vi "Limelight HatchPanel.vi"(7 "Max Speed":dbl=0.6, 8 "error in":errorcluster, 10 "Max Time ms (2000)":u32=2000, 11 "Min time ms (500)":u32=500) -> (0 "error out":errorcluster, 3 "Timed Out?":bool)   [LabVIEW 2018]
uses:
  <vilib>/Rock Robotics/Network Tables/NT Read Number.vi
  Auton Kill Switch.vi
panel:
  in  "allowed error":dbl=2.5
  in  "kpDist":dbl=0.2
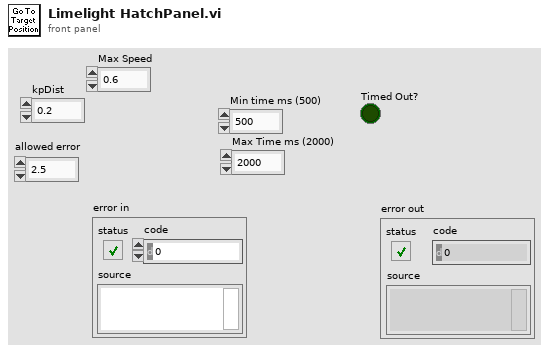
[diagram p1: front panel]
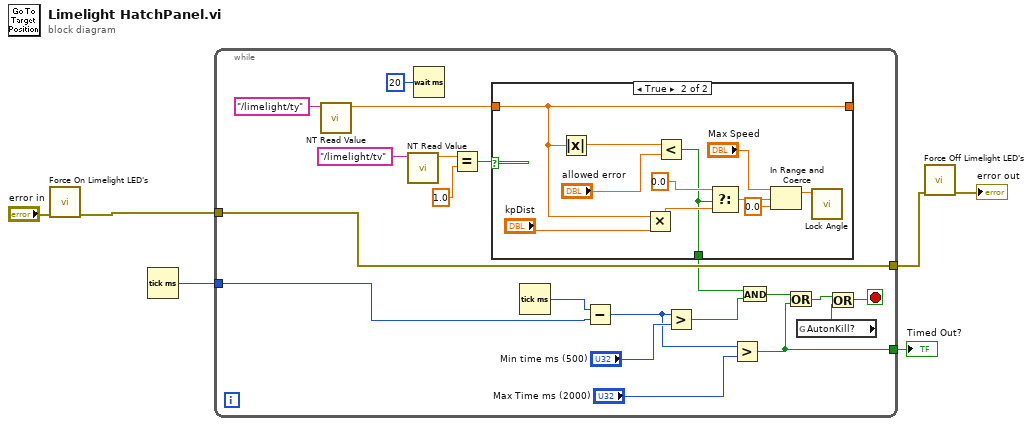
[diagram p0: block diagram]
diagram:
  n1 = call "Force On Limelight LED's.vi"("error in"="error in") -> ("error out"=w5:errorcluster)  [unwired: 9 in]
  n2 = Tick Count (ms)() -> (millisecond timer value=w2:u32)
  n3 = while {
    tunnel: w5 -> [w19]
    tunnel: [w19] -> w4
    tunnel: w2 -> [w17]
    tunnel: [w9] -> w1
    stop <- w8 stop-if-true
    n4 = call-poly <vilib>:"NT Read Value.vi"("Name"="/limelight/ty") -> ("Numeric"=w21:dbl)  [unwired: 9 in, 1 out]
    n5 = call-poly <vilib>:"NT Read Value.vi"("Name"="/limelight/tv") -> ("Numeric"=w25:dbl)  [unwired: 9 in, 1 out]
    n6 = Wait (ms)(milliseconds to wait=u32 20) -> ()  [unwired: 1 out]
    n7 = Equal?(x=w25, y=1.0) -> (x = y?=w23:bool)
    n8 = case shown="True" w23 {
      tunnel: [w27 w37] -> _
      tunnel: w21 -> [w27 w37]
      tunnel: [_ w32] -> w16
      frame False {
      }
      frame True {
        n9 = Absolute Value(x=w37) -> (abs(x)=w36:dbl)
        n10 = Multiply(x=w37, y="kpDist") -> (x*y=w34:dbl)
        n11 = Less?(x=w36, y="allowed error") -> (x < y?=w32:bool)
        n12 = Select(t=0.0, s=w32, f=w34) -> (s? t:f=w30:dbl)
        n13 = In Range and Coerce(upper limit="Max Speed", x=w30, lower limit=0.0) -> (coerced(x)=w31:dbl)  [unwired: 1 out]
        n14 = call "Lock Angle.vi"("Setpoint"=w31) -> ()  [unwired: 11 in]
      }
    }
    n15 = Tick Count (ms)() -> (millisecond timer value=w18:u32)
    n16 = Subtract(x=w18, y=w17) -> (x-y=w11:u32)
    n17 = Greater?(x=w11, y="Min time ms (500)") -> (0:w14:bool)
    n18 = Greater?(x=w11, y="Max Time ms (2000)") -> (0:w9:bool)
    n19 = And(x=w16, y=w14) -> (x .and. y?=w13:bool)
    n20 = Or(x=w13, y=w9) -> (x .or. y?=w12:bool)
    n21 = global read "Auton Kill Switch.vi" "AutonKill?"() -> (w7:bool)
    n22 = Or(x=w12, y=w7) -> (x .or. y?=w8:bool)
  }
  "Timed Out?" <- w1
  n23 = call "Force Off Limelight LED's.vi"("error in"=w4) -> ("error out"=→"error out":errorcluster)  [unwired: 9 in]
